vi "Stiffness Test.vi"() -> ()   [LabVIEW 2016]
uses:
  Test Actuator State.lvclass
  Model/Model/Model.lvclass
  <vilib>/Platform/TimedLoop/XDataNode/timing_clust.ctl
  <vilib>/Platform/TimedLoop/XDataNode/nitl_modes.ctl
  <vilib>/Platform/TimedLoop/XDataNode/wakeup.ctl
  Typedefs/TestStatus.ctl
  Model/Model/Model.lvclass/Model.ctl
  <vilib>/platform/TimedLoop/XDataNode/XDataNode.xnode
  <vilib>/Platform/TimedLoop/XDataNode/XDNodeRunTimeDep.lvlib
  Typedefs/HPMT_Typedefs.lvlib
panel:
  out "Test Actuator State out":refnum<class "Test Actuator State.lvclass">
  out "Model out":refnum<class "Model.lvclass">
  out "error out":errorcluster
  in  "error in (no error)":errorcluster
  in  "Model in":refnum<class "Model.lvclass">
  in  "Test Actuator State in":refnum<class "Test Actuator State.lvclass">
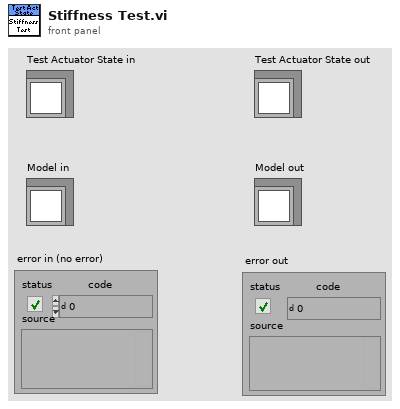
[diagram p1: front panel]
types:
  T1 = typedef "HPMT_Typedefs.lvlib/TestStatus.ctl" = enum16{"Not Run", "Running", "Passed", "Failed"}
  T2 = typedef "HPMT_Typedefs.lvlib/AllTestStatus.ctl" = cluster{"Stiffness Test":T1}
  T3 = typedef "XDNodeRunTimeDep.lvlib/timing_clust.ctl" = cluster{"Expected End [f-1]":u64, "Actual End [f-1]":u64, "Finished Late? [f-1]":bool, "Expected End [i-1]":u64, "Actual End [i-1]":u64, "Finished Late? [i-1]":bool, "Expected Start [i]":u64, "Actual Start [i]":u64, "Expected Start [f]":u64, "Actual Start [f]":u64, "Source Name":string, "Structure Name":string, "Period":i64, "Deadline":i64, "Offset":i64, "Start":i64, "Priority":i32, "Timeout":i32, "Mode":T4, "Wakeup Reason":T5, "Error":errorcluster, "Source Type":string, "Secondary Source Type":string, "Global End Time":u64, "Global Start Time":u64, "Frame Duration":u64, "Iteration Duration":u64, "Assigned CPU":i32, "I/O Scan Engine Mode":u32}
  T4 = typedef "XDNodeRunTimeDep.lvlib/nitl_modes.ctl" = enum32{"No Change", "Process missed periods, maintain original phase", "Discard missed periods, maintain original phase", "Process missed periods, ignore original phase", "Discard missed periods, ignore original phase"}
  T5 = typedef "XDNodeRunTimeDep.lvlib/wakeup.ctl" = enum32{"Normal", "Aborted", "Asynchronous wakeup", "Timing source error", "Timed loop error", "Timeout"}
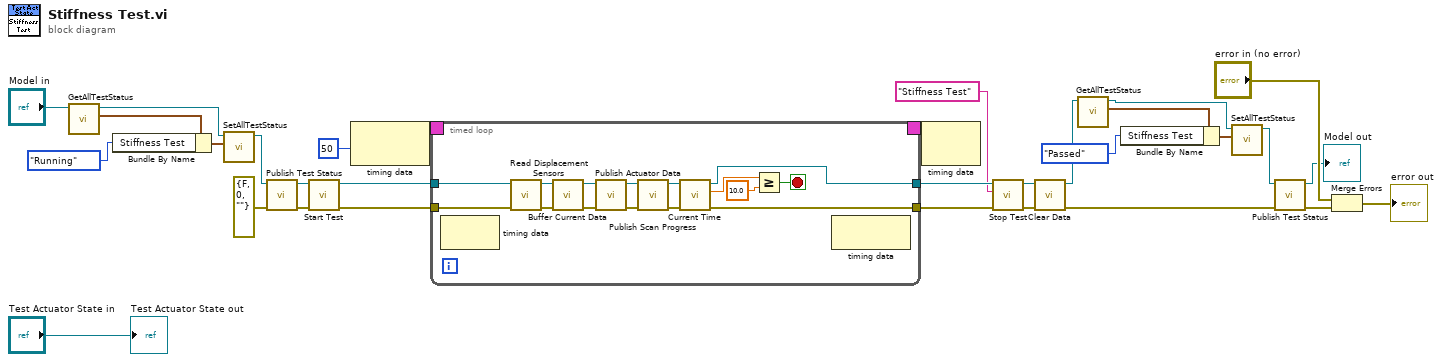
[diagram p0: block diagram]
diagram:
  n1 = call "GetAllTestStatus.vi"("Model in"="Model in") -> ("AllTestStatus"=w29:T2, "Model out"=w27:refnum<class "Model.lvclass">)  [unwired: 9 in]
  n2 = Bundle By Name(cluster=w29, "Stiffness Test"=TestStatus."Running" ("TestStatus")) -> (w28:T2)
  n3 = call "SetAllTestStatus.vi"("AllTestStatus"=w28, "Model in"=w27) -> ("Model out"=w26:refnum<class "Model.lvclass">)  [unwired: 9 in]
  n4 = call "Publish Test Status.vi"("error in (no error)"=errorcluster {"status"=FALSE, "code"=0, "source"=""} ("error constant"), "Model in"=w26) -> ("error out"=w24:errorcluster, "Model out"=w23:refnum<class "Model.lvclass">)  [unwired: 8 in]
  n5 = call "Start Test.vi"("error in (no error)"=w24, "Model in"=w23) -> ("error out"=w18:errorcluster, "Model out"=w19:refnum<class "Model.lvclass">)  [unwired: 8 in]
  n6 = node-c288(50) -> (w22:T3)
  n7 = timed-loop {
    timing: w22 -> [_]
    timing-out: [_] -> w21
    tunnel: w19 -> [w39]
    tunnel: w18 -> [w37]
    tunnel: [w41] -> w15
    tunnel: [w40] -> w14
    stop <- w44 stop-if-true
    n8 = node-c288() -> ()  [unwired: 1 in, 1 out]
    n9 = call "Read Displacement Sensors.vi"("error in (no error)"=w37, "Model in"=w39) -> ("error out"=w34:errorcluster, "Model out"=w35:refnum<class "Model.lvclass">)  [unwired: 8 in]
    n10 = call "Buffer Current Data.vi"("error in (no error)"=w34, "Model in"=w35) -> ("error out"=w32:errorcluster, "Model out"=w33:refnum<class "Model.lvclass">)  [unwired: 8 in]
    n11 = call "Publish Actuator Data.vi"("error in (no error)"=w32, "Model in"=w33) -> ("error out"=w36:errorcluster, "Model out"=w38:refnum<class "Model.lvclass">)  [unwired: 8 in]
    n12 = call "Publish Scan Progress.vi"("error in (no error)"=w36, "Model in"=w38) -> ("error out"=w43:errorcluster, "Model out"=w42:refnum<class "Model.lvclass">)  [unwired: 8 in]
    n13 = call "Current Time.vi"("error in (no error)"=w43, "Model in"=w42) -> ("error out"=w40:errorcluster, "Time"=w45:dbl, "Model out"=w41:refnum<class "Model.lvclass">)  [unwired: 7 in]
    n14 = Greater Or Equal?(x=w45, y=10.0) -> (x >= y?=w44:bool)
    n15 = node-c288() -> ()  [unwired: 1 in, 1 out]
  }
  n16 = node-c288(w21) -> ()  [unwired: 1 out]
  n17 = call "Stop Test.vi"("error in (no error)"=w14, "Test"="Stiffness Test", "Model in"=w15) -> ("error out"=w17:errorcluster, "Model out"=w16:refnum<class "Model.lvclass">)  [unwired: 7 in]
  n18 = call "Clear Data.vi"("error in (no error)"=w17, "Model in"=w16) -> ("error out"=w10:errorcluster, "Model out"=w7:refnum<class "Model.lvclass">)  [unwired: 8 in]
  n19 = call "GetAllTestStatus.vi"("Model in"=w7) -> ("AllTestStatus"=w6:T2, "Model out"=w4:refnum<class "Model.lvclass">)  [unwired: 9 in]
  n20 = Bundle By Name(cluster=w6, "Stiffness Test"=TestStatus."Passed" ("TestStatus")) -> (w5:T2)
  n21 = call "SetAllTestStatus.vi"("AllTestStatus"=w5, "Model in"=w4) -> ("Model out"=w9:refnum<class "Model.lvclass">)  [unwired: 9 in]
  n22 = call "Publish Test Status.vi"("error in (no error)"=w10, "Model in"=w9) -> ("error out"=w11:errorcluster, "Model out"=→"Model out":refnum<class "Model.lvclass">)  [unwired: 8 in]
  n23 = Merge Errors("error in (no error)", w11) -> (→"error out":errorcluster)
  "Test Actuator State out" <- "Test Actuator State in"
